vi "DrawNamePic.vi"(11 "mu08ArrayIn":u8[](array[numeric])) -> (3 "NamePic":picture)   [LabVIEW 2011]
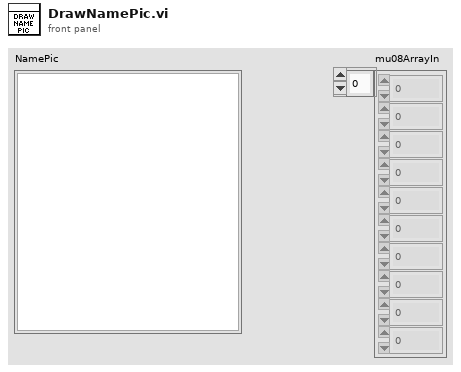
[diagram p1: front panel]
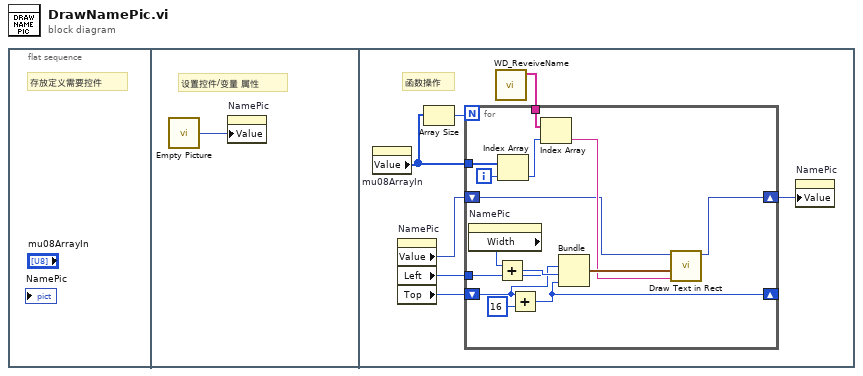
[diagram p0: block diagram]
diagram:
  n1 = flat-sequence {
    frame #0 {
      # "存放定义需要控件"
    }
    frame #1 {
      # "设置控件/变量 属性"
      n2 = call "Empty Picture"() -> ("empty picture"=w1:picture)
      n3 = property on="NamePic" class="Pict"("Value"=w1) -> ()  [unwired: 2 in, 2 out]
    }
    frame #2 {
      # "函数操作"
      n4 = property on="mu08ArrayIn" class="Arr (严格)"() -> ("Value"=w4:u8[])  [unwired: 2 in, 2 out]
      n5 = property on="NamePic" class="Pict"() -> ("Value"=w2:picture, "Left"=w6:i32, "Top"=w7:i32)  [unwired: 2 in, 2 out]
      n6 = Array Size(array=w4) -> (size(s)=w3:i32)
      n7 = call "WD_ReveiveName.vi"() -> ("ArrayOut"=w5:string[])  [unwired: 11 in]
      n8 = for {
        N: w3 -> [_]
        tunnel: w4 -> [w22]
        tunnel: w5 -> [w20]
        shift-right: [w9] -> _
        shift-left: w7 -> [w15]
        shift-right: [w10] -> w8
        shift-left: w2 -> [w11]
        tunnel: w6 -> [w14]
        i -> [w21]
        n9 = property on="NamePic" class="Pict"() -> ("Width"=w17:u32)  [unwired: 2 in, 2 out]
        n10 = Add(x=w17, y=w14) -> (x+y=w16:u32)
        n11 = Index Array(array=w22, index=w21) -> (element=w19:u8)
        n12 = Add(x=w15, y=16) -> (x+y=w9:i32)
        n13 = Index Array(array=w20, index=w19) -> (element=w12:string)
        n14 = Bundle("Left"=w14, "Top"=w15, w16, w9) -> (w13:cluster{"Left":i32, "Top":i32, u32, i32})  [unwired: 1 in]
        n15 = call <vilib>:"Draw Text in Rect.vi"("text"=w12, "rect"=w13, "picture"=w11) -> ("new picture"=w10:picture)  [unwired: 8 in]
      }
      n16 = property on="NamePic" class="Pict"("Value"=w8) -> ()  [unwired: 2 in, 2 out]
    }
  }
